vi "dft_normalizada.vi"(10 "FFT size":i32, 11 "X":dbl[](array[numeric])) -> (2 "Escalado eje":dbl, 3 "DFT X":dbl[](array[numeric]))   [LabVIEW 2020]
uses:
  <vilib>/Analysis/2dsp.llb/Real FFT.vi
  <vilib>/Analysis/NI_AALPro.lvlib
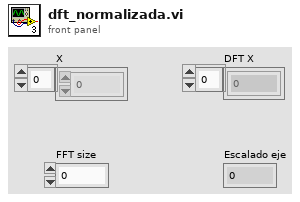
[diagram p1: front panel]
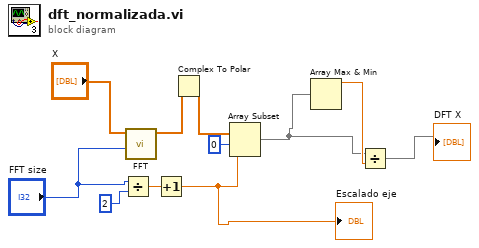
[diagram p0: block diagram]
diagram:
  n1 = Divide(x="FFT size", y=2) -> (x/y=w10:dbl)
  n2 = call-poly <vilib>:"FFT.vi"("FFT size"="FFT size", "X"="X") -> ("FFT {X}"=w7:cdb[])  [unwired: 8 in, 1 out]
  n3 = Increment(x=w10) -> (x+1=w1:dbl)
  "Escalado eje" <- w1
  n4 = Complex To Polar(r * e^(i*theta)=w7) -> (r=w6:dbl[])  [unwired: 1 out]
  n5 = Array Subset(array=w6, index=0, length=w1) -> (w4:dbl[])
  n6 = Array Max & Min(array=w4) -> (max value=w5:dbl)  [unwired: 3 out]
  n7 = Divide(x=w4, y=w5) -> (x/y=→"DFT X":dbl[])
